vi "LineEquationTO2points.vi"(1 "Line Equation":cluster{"A":dbl, "B":dbl, "C":dbl}) -> (0 "Line 2":T1)   [LabVIEW 2016]
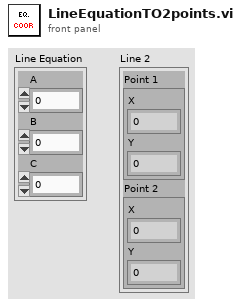
[diagram p1: front panel]
types:
  T1 = cluster{"Point 1":cluster{"X":sgl, "Y":sgl}, "Point 2":cluster{"X":sgl, "Y":sgl}}
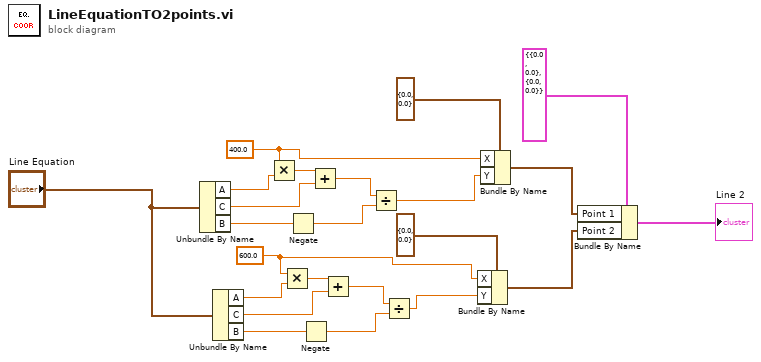
[diagram p0: block diagram]
diagram:
  w17 = 600.0
  w15 = 400.0
  n1 = Unbundle By Name("Line Equation") -> ("A"=w1:dbl, "C"=w3:dbl, "B"=w5:dbl)
  n2 = Unbundle By Name("Line Equation") -> ("A"=w12:dbl, "C"=w10:dbl, "B"=w8:dbl)
  n3 = Multiply(x=w15, y=w1) -> (x*y=w2:dbl)
  n4 = Multiply(x=w17, y=w12) -> (x*y=w11:dbl)
  n5 = Negate(x=w5) -> (-x=w6:dbl)
  n6 = Negate(x=w8) -> (-x=w7:dbl)
  n7 = Add(x=w2, y=w3) -> (x+y=w4:dbl)
  n8 = Add(x=w11, y=w10) -> (x+y=w9:dbl)
  n9 = Divide(x=w4, y=w6) -> (x/y=w16:dbl)
  n10 = Divide(x=w9, y=w7) -> (x/y=w19:dbl)
  n11 = Bundle By Name(cluster=cluster{"X":sgl, "Y":sgl} {"X"=0.0, "Y"=0.0} ("Point 1"), "X"=w17, "Y"=w19) -> (w22:cluster{"X":sgl, "Y":sgl})
  n12 = Bundle By Name(cluster=cluster{"X":sgl, "Y":sgl} {"X"=0.0, "Y"=0.0} ("Point 1"), "X"=w15, "Y"=w16) -> (w21:cluster{"X":sgl, "Y":sgl})
  n13 = Bundle By Name(cluster=T1 {"Point 1"={"X"=0.0, "Y"=0.0}, "Point 2"={"X"=0.0, "Y"=0.0}} ("Line 2"), "Point 1"=w21, "Point 2"=w22) -> (→"Line 2":T1)
